vi "Unmarshal.vi"(8 "error in (no error)":errorcluster, 10 "Buffer":u8[](array[numeric]), 11 "int32 in":refnum<class "int32.lvclass">) -> (0 "error out":errorcluster, 2 "Buffer Count":i32=8, 3 "int32 out":refnum<class "int32.lvclass">)   [LabVIEW 2020, in "Protobuf RAW.lvlib" / "int32.lvclass"]
uses:
  int32.lvclass
  int32.lvclass/int32.ctl
  Protobuf RAW.lvlib
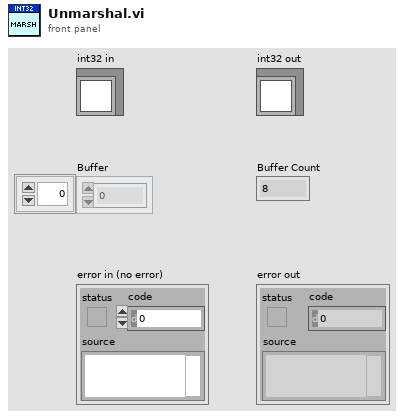
[diagram p1: front panel]
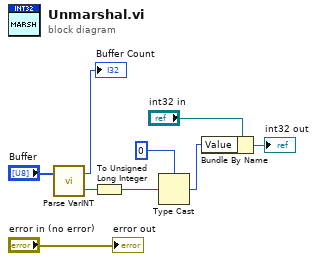
[diagram p0: block diagram]
diagram:
  n1 = call "Parse VarINT.vi"("Buffer"="Buffer") -> ("Numeric"=w5:u64, "Bytes"=→"Buffer Count":i32)  [unwired: 1 in]
  n2 = To Unsigned Long Integer(number=w5) -> (unsigned 32bit integer=w1:u32)
  n3 = Type Cast(type=0 ("Numeric"), x=w1) -> (*(type *) &x=w4:i32)
  n4 = Bundle By Name(cluster="int32 in", "Value"=w4) -> (→"int32 out":refnum<class "int32.lvclass">)
  "error out" <- "error in (no error)"
